vi "GetLogFileArray.vi"(8 "error in (no error)":errorcluster) -> (0 "error out":errorcluster, 2 "LogFileNumber":u32, 3 "LogFileArray":path[](array[path]))   [LabVIEW 2011]
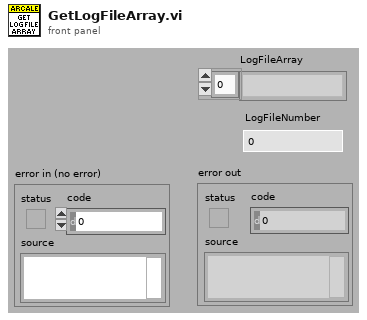
[diagram p1: front panel]
types:
  T1 = typedef "ApplicationPaths.ctl" = cluster{"Data Path":path, "Log Path":path, "Tmp Path":path}
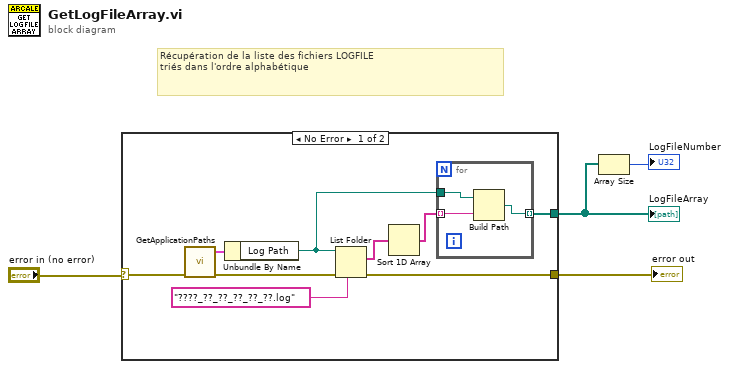
[diagram p0: block diagram]
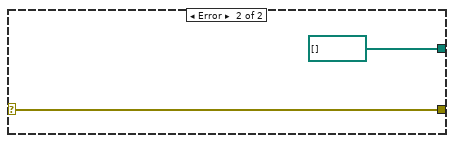
[diagram p2: hidden frame]
diagram:
  # "Récupération de la liste des fichiers LOGFILE \ntriés dans l'ordre alphabétique"
  n1 = case shown="No Error" "error in (no error)" {
    selector: "error in (no error)" -> [w13 w18]
    tunnel: [w9 w18] -> w3
    tunnel: [w5 path[] []] -> w2
    frame No Error {
      n2 = call "GetApplicationPaths.vi"("error in (no error)"=w13) -> ("error out"=w12:errorcluster, "ApplicationPath"=w11:T1)  [unwired: 9 in]
      n3 = Unbundle By Name(w11) -> ("Log Path"=w8:path)
      n4 = List Folder(path=w8, pattern="????_??_??_??_??_??.log", error in=w12) -> (filenames=w7:string[], error out=w9:errorcluster)  [unwired: 1 in, 2 out]
      n5 = Sort 1D Array(array=w7) -> (sorted array=w6:string[])
      n6 = for {
        tunnel: w6 -> [w15] mode=indexing
        tunnel: w8 -> [w16]
        tunnel: [w14] -> w5 mode=indexing
        n7 = Build Path(base path=w16, name or relative path=w15) -> (appended path=w14:path)
      }
    }
    frame Error {
    }
  }
  "error out" <- w3
  "LogFileArray" <- w2
  n8 = Array Size(array=w2) -> (size(s)=→"LogFileNumber":i32)
